vi "INI_RS232_Appl.vi"(0 "Device INI Config File Path":path=path "D:/LABVIEW/Examples/INI Devices/DeviceConfig.ini", 2 "MListBox Row":u16=2 max=8, 7 "MCListbox Ref":refnum<vi>) -> (6 "COM Port":refnum<visa-resource-name>, 8 "Dev OK":bool, 9 "Handle":u32, 10 "error out":errorcluster)   [LabVIEW 2018]
uses:
  <vilib>/Utility/miscctls.llb/LVRowAndColumnTypeDef.ctl
  <vilib>/Utility/config.llb/Read Key (String).vi
  <vilib>/Utility/config.llb/NI_LVConfig.lvlib
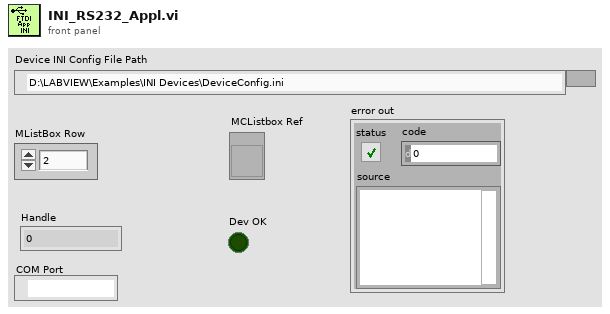
[diagram p1: front panel]
types:
  T1 = typedef "LVRowAndColumnTypeDef.ctl" = cluster{"Row":i32, "Column":i32}
  T2 = typedef "NI_LVConfig.lvlib/Config Data RefNum.ctl" = refnum<k1>
  T3 = cluster{"Type":u32, "VID":string, "PID":string, "Serial Number":string, "Description":string}
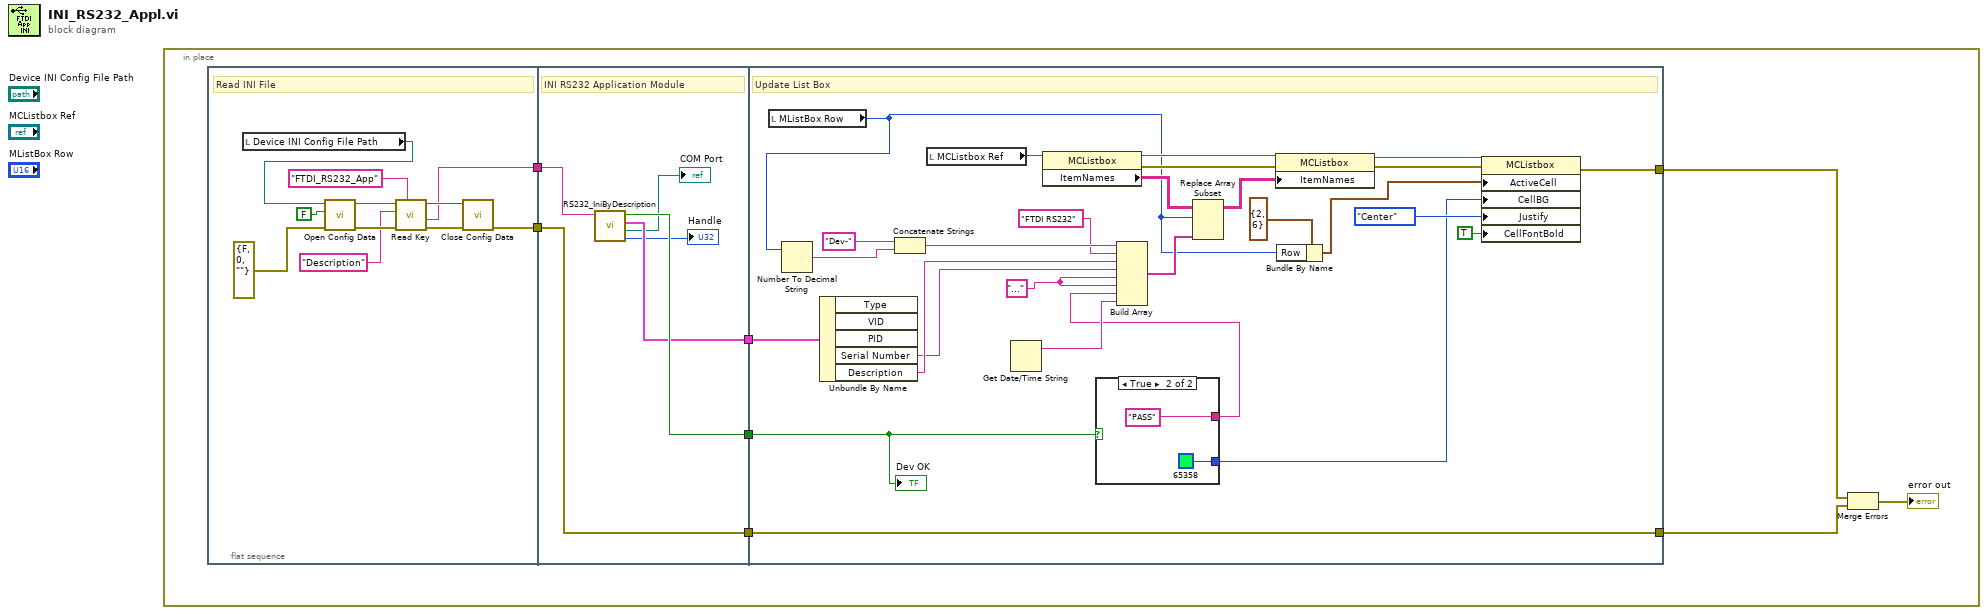
[diagram p0: block diagram]
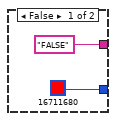
[diagram p2: hidden frame]
diagram:
  n1 = in-place {
    n2 = flat-sequence {
      tunnel: [w12] -> w8
      tunnel: [w9] -> w3
      tunnel: w8 -> [w25]
      tunnel: [w25] -> w6
      tunnel: w3 -> [w24]
      tunnel: [w23] -> w2
      tunnel: [w22] -> w1
      tunnel: [w39] -> w7
      tunnel: [w38] -> w5
      tunnel: w6 -> [w38]
      tunnel: w2 -> [w26]
      tunnel: w1 -> [w30]
      frame #0 {
        # "Read INI File"
        n3 = local read "Device INI Config File Path"() -> (w14:path)
        n4 = call <vilib>:"Open Config Data.vi"("error in (no error)"=errorcluster {"status"=FALSE, "code"=0, "source"=""} ("error constant"), "create file if necessary (T)"=FALSE, "configuration file path"=w14) -> ("error out"=w17:errorcluster, "refnum"=w18:T2)  [unwired: 6 in, 1 out]
        n5 = call-poly <vilib>:"Read Key.vi"("section"="FTDI_RS232_App", "error in (no error)"=w17, "key"="Description", "refnum"=w18) -> ("error out"=w11:errorcluster, "value"=w9:string, "refnum out"=w10:T2)  [unwired: 4 in, 1 out]
        n6 = call <vilib>:"Close Config Data.vi"("error in (no error)"=w11, "refnum"=w10) -> ("error out"=w12:errorcluster)  [unwired: 8 in, 1 out]
      }
      frame #1 {
        # "INI RS232 Application Module"
        n7 = call "RS232_IniByDescription.vi"("Description"=w24) -> ("Handle"=→"Handle":u32, "COM Port"=→"COM Port":refnum<visa-resource-name>, "Device Information"=w22:T3, "Ok?"=w23:bool)  [unwired: 7 in]
      }
      frame #2 {
        w27 = "..."
        # "Update List Box"
        n8 = local read "MListBox Row"() -> (w32:u16)
        n9 = Number To Decimal String(number=w32) -> (decimal integer string=w35:string)  [unwired: 1 in]
        n10 = Unbundle By Name(w30) -> ("Serial Number"=w28:string, "Description"=w29:string)  [unwired: 3 out]
        n11 = Concatenate Strings("Dev-", w35) -> (w34:string)
        n12 = local read "MCListbox Ref"() -> (w33:refnum<vi>)
        n13 = Get Date/Time String() -> (date string=w44:string)  [unwired: 3 in, 1 out]
        n14 = property class="MCListbox"(reference=w33) -> (reference out=w46:refnum<vi>, error out=w47:errorcluster, "ItemNames"=w48:string[][])  [unwired: 1 in]
        n15 = case shown="True" w26 {
          tunnel: [u32 16711680 u32 65358] -> w41
          tunnel: ["FALSE" ("element") "PASS" ("element")] -> w40
          frame False {
          }
          frame True {
          }
        }
        n16 = Build Array(w34, "FTDI RS232", w29, w28, w27, w27, w40, w44) -> (w50:string[])
        n17 = Replace Array Subset(array=w48, new element=w50, index (row)=w32) -> (w49:string[][])  [unwired: 1 in]
        n18 = property class="MCListbox"(reference=w46, error in=w47, "ItemNames"=w49) -> (reference out=w51:refnum<vi>, error out=w52:errorcluster)
        n19 = Bundle By Name(cluster=T1 {"Row"=2, "Column"=6} ("Active Cell:Active Cell"), "Row"=w32) -> (w42:T1)
        n20 = property class="MCListbox"(reference=w51, error in=w52, "ActiveCell"=w42, "CellBG"=w41, "Justify"=enum16{"Left", "Center", "Right"}."Center" ("Active Cell:Cell Justification"), "CellFontBold"=TRUE ("Active Cell:Cell Font:Bold")) -> (error out=w39:errorcluster)  [unwired: 1 out]
        "Dev OK" <- w26
      }
    }
    n21 = Merge Errors(w7, w5) -> (→"error out":errorcluster)
  }
